vi "模板-多副本重入异步调用-(不可运行).vi"() -> ()   [LabVIEW 2013]
panel:
  out "重入VI控件引用数组":refnum<vi>[](array[refnum])
  out "VI引用数组":refnum<vi>[](array[refnum])
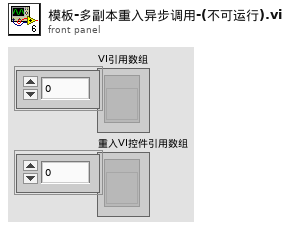
[diagram p1: front panel]
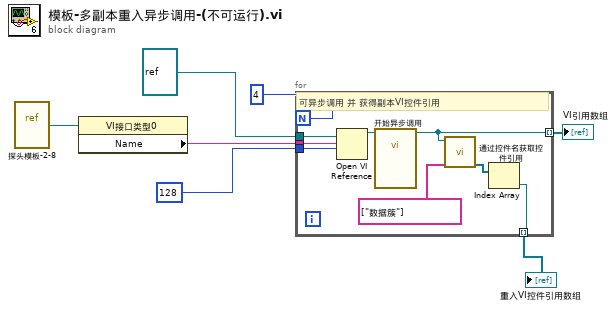
[diagram p0: block diagram]
diagram:
  n1 = vi-ref "探头模板-2-8.vi"() -> (w3:refnum<vi>)
  n2 = property class="VI接口类型0"(reference=w3) -> ("Name"=w4:string)  [unwired: 1 in, 2 out]
  n3 = for {
    N: 4 -> [_]
    tunnel: w4 -> [w15]
    tunnel: 128 ("选项") -> [w14]
    tunnel: refnum<vi> refnum ("类型说明符VI引用句柄（仅用于类型）") -> [w13]
    tunnel: [w8] -> w2 mode=indexing
    tunnel: [w9] -> w1 mode=indexing
    # "可异步调用 并 获得副本VI控件引用"
    n4 = Open VI Reference(type specifier VI Refnum (for type only)=w13, vi path=w15, options=w14) -> (vi reference=w10:refnum<vi>)  [unwired: 3 in, 1 out]
    n5 = call-by-ref "开始异步调用"(reference=w10) -> (reference out=w8:refnum<vi>)  [unwired: 13 in, 1 out]
    n6 = call "通过控件名获取控件引用.vi"("控件名数组"=string[] ["数据簇"], "VI引用"=w8) -> ("控件引用输出"=w12:refnum<vi>[])  [unwired: 9 in]
    n7 = Index Array(array=w12) -> (element=w9:refnum<vi>)  [unwired: 1 in]
  }
  "VI引用数组" <- w2
  "重入VI控件引用数组" <- w1
